vi "connect.vi"(6 "ms timeout (10000)":i32=10000, 8 "error in (no error)":errorcluster, 9 "auth":T2={"user"="user", "password"="rOprNGfwEbeRWgbNEkqO"}, 10 "port (28015)":u16=28015, 11 "host (\"localhost\")":string="localhost") -> (0 "error out":errorcluster, 2 "server_signature":string, 3 "rethinkdb":refnum<class "rethinkdb.lvclass">)   [LabVIEW 2017, in "rethinkdb.lvclass"]
uses:
  rethinkdb.lvclass
  b554cd97-6ca4-476d-9024-a4695d90b2fb.vi
  msg/rethinkdb_msg_connect_auth.ctl
  rethinkdb_settings.ctl
panel:
  in  "settings":T1
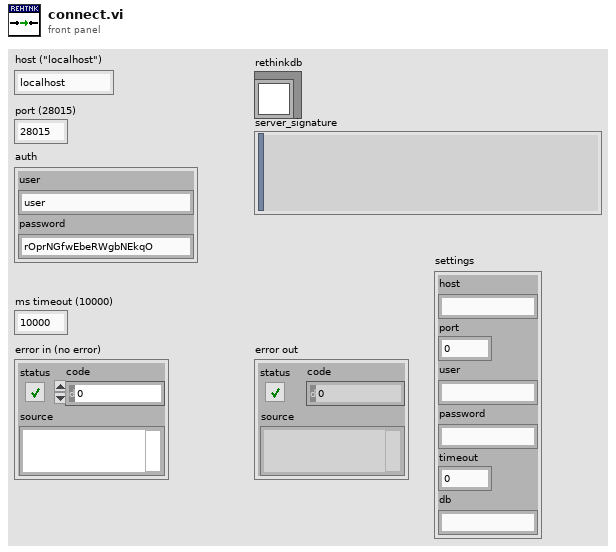
[diagram p1: front panel]
types:
  T1 = typedef "rethinkdb_settings.ctl" = cluster{"host":string, "port":u16, "user":string, "password":string, "timeout":i32, "db":string}
  T2 = typedef "rethinkdb_msg_connect_auth.ctl" = cluster{"user":string, "password":string}
  T3 = typedef "json_element.ctl" = cluster{"path":string, "type":T4, "value":variant}
  T4 = typedef "json_element_type.ctl" = enum8{"null", "bool", "int", "uint", "float", "string", "array", "object"}
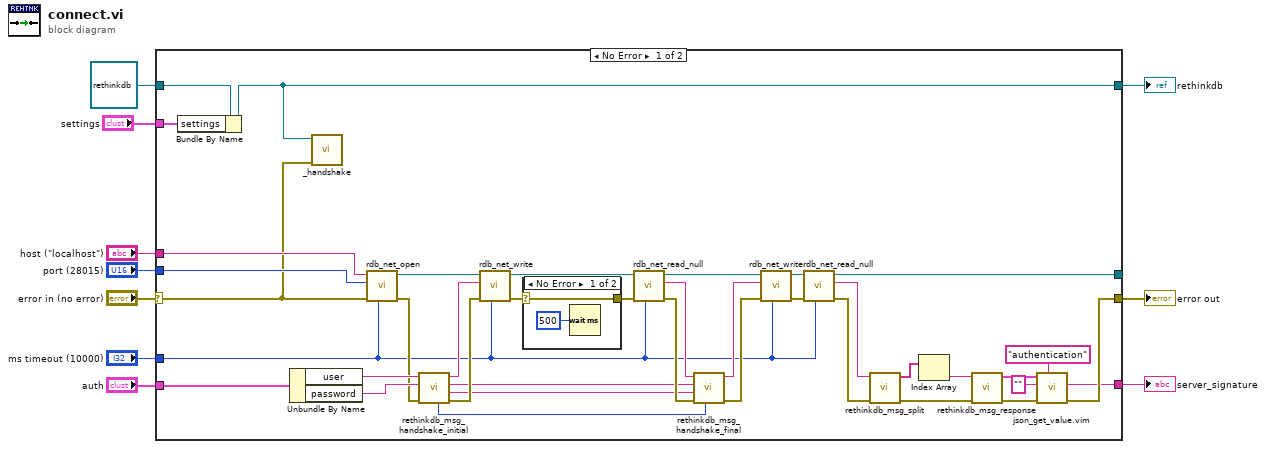
[diagram p0: block diagram]
diagram:
  n1 = case shown="No Error" "error in (no error)" {
    selector: "error in (no error)" -> [w12 w54]
    tunnel: "host (\"localhost\")" -> [w16 _]
    tunnel: "port (28015)" -> [w15 _]
    tunnel: "ms timeout (10000)" -> [w17 _]
    tunnel: [w26 w54] -> w6
    tunnel: [w34 _] -> _
    tunnel: "auth" -> [w49 _]
    tunnel: [w25 _] -> w4
    tunnel: [w11 w53] -> w3
    tunnel: refnum<class "rethinkdb.lvclass"> refnum ("rethinkdb") -> [w14 w53]
    tunnel: "settings" -> [w13 _]
    frame No Error {
      n2 = Bundle By Name(cluster=w14, "settings"=w13) -> (w11:refnum<class "rethinkdb.lvclass">)
      n3 = Unbundle By Name(w49) -> ("user"=w48:string, "password"=w47:string)
      n4 = call "_handshake.vi"("error in (no error)"=w12, "rethinkdb in"=w11) -> ()  [unwired: 8 in, 2 out]
      n5 = call "rdb_net_open.vi"("timeout ms (10000)"=w17, "error in (no error)"=w12, "port (28015)"=w15, "host (\"localhost\")"=w16) -> ("error out"=w19:errorcluster, "conn out"=w18:refnum<k5>)  [unwired: 6 in]
      n6 = call "rethinkdb_msg_handshake_initial.vi"("error in (no error)"=w19, "password"=w47, "user"=w48) -> ("error out"=w45:errorcluster, "client_first_message"=w32:string, "dup password"=w33:string, "initial_message"=w44:string, "protocol_version"=w31:i32)  [unwired: 4 in]
      n7 = call "rdb_net_write.vi"("timeout ms (10000)"=w17, "error in (no error)"=w45, "data in"=w44, "conn in"=w18) -> ("error out"=w37:errorcluster, "conn out"=w46:refnum<k5>)  [unwired: 5 in, 1 out]
      n8 = case shown="No Error" w37 {
        selector: w37 -> [w50 w52]
        tunnel: [w50 w52] -> w38
        frame No Error {
          n9 = Wait (ms)(milliseconds to wait=u32 500) -> ()  [unwired: 1 out]
        }
        frame Error {
        }
      }
      n10 = call "rdb_net_read_null.vi"("timeout ms (10000)"=w17, "error in (no error)"=w38, "conn in"=w46) -> ("error out"=w41:errorcluster, "data out"=w39:string, "conn out"=w42:refnum<k5>)  [unwired: 6 in]
      n11 = call "rethinkdb_msg_handshake_final.vi"("protocol_version"=w31, "error in (no error)"=w41, "client_first_message"=w32, "password"=w33, "server_response (json)"=w39) -> ("error out"=w40:errorcluster, "authentication_request"=w36:string)  [unwired: 5 in]
      n12 = call "rdb_net_write.vi"("timeout ms (10000)"=w17, "error in (no error)"=w40, "data in"=w36, "conn in"=w42) -> ("error out"=w35:errorcluster, "conn out"=w43:refnum<k5>)  [unwired: 5 in, 1 out]
      n13 = call "rdb_net_read_null.vi"("timeout ms (10000)"=w17, "error in (no error)"=w35, "conn in"=w43) -> ("error out"=w24:errorcluster, "data out"=w22:string, "conn out"=w34:refnum<k5>)  [unwired: 6 in]
      n14 = call "rethinkdb_msg_split.vi"("error in (no error)"=w24, "data in"=w22) -> ("error out"=w23:errorcluster, "messages"=w21:string[])  [unwired: 7 in, 1 out]
      n15 = Index Array(array=w21) -> (element=w20:string)  [unwired: 1 in]
      n16 = call "rethinkdb_msg_response.vi"("error in (no error)"=w23, "response"=w20) -> ("error out"=w30:errorcluster, "elements"=w29:T3[])  [unwired: 8 in]
      n17 = call "json_get_value.vim"("key"="authentication", "error in (no error)"=w30, "default"="", "elements in"=w29) -> ("error out"=w26:errorcluster, "value"=w25:string)  [unwired: 4 in, 2 out]
    }
    frame Error {
    }
  }
  "error out" <- w6
  "rethinkdb" <- w3
  "server_signature" <- w4
